vi "spring - defer panel updates.vi"(7 "tree ref":refnum<vi>, 8 "error in (no error) (will be ignored)":errorcluster, 10 "defer panel updates":bool) -> (0 "error out":errorcluster)   [LabVIEW 2014]
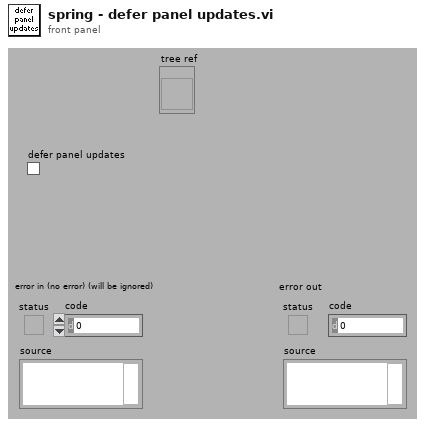
[diagram p1: front panel]
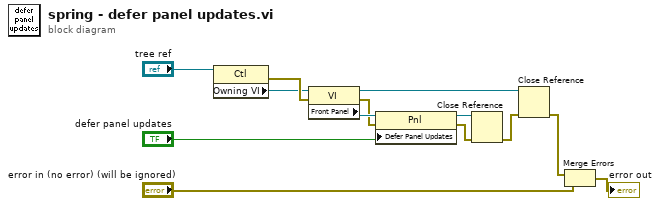
[diagram p0: block diagram]
diagram:
  n1 = property class="Ctl"(reference="tree ref") -> (error out=w12:errorcluster, "Owning VI"=w11:refnum<vi>)  [unwired: 1 in, 1 out]
  n2 = property class="VI"(reference=w11, error in=w12) -> (reference out=w10:refnum<vi>, error out=w8:errorcluster, "Front Panel"=w9:refnum<vi>)
  n3 = property class="Pnl"(reference=w9, error in=w8, "Defer Panel Updates"="defer panel updates") -> (reference out=w7:refnum<vi>, error out=w6:errorcluster)
  n4 = Close Reference(reference=w7, error in (no error)=w6) -> (error out=w5:errorcluster)
  n5 = Close Reference(reference=w10, error in (no error)=w5) -> (error out=w3:errorcluster)
  n6 = Merge Errors(w3, "error in (no error) (will be ignored)") -> (→"error out":errorcluster)
